vi "Keithley 6514 Limits Config.vi"(0 "Resource In":refnum<visa-resource-name>, 1 "limit 1 test (off:F)":bool, 2 "limit 2 test (off:F)":bool, 3 "Input Path for Limits (Inputs:0)":u16(ring) items=["Inputs ", "Results of Math"], 4 "pass line":dbl min=0.0 max=15.0 step=1.0, 5 "error in (no error)":T1, 6 "upper limit 1 (1)":dbl=1.0 min=-9.99999e+20 max=9.99999e+20 step=1.0 format="%.5e", 7 "upper limit 2 (1)":dbl=1.0 min=-9.99999e+20 max=9.99999e+20 step=1.0 format="%.5e", 8 "lower limit 1 (-1)":dbl=-1.0 min=-9.99999e+20 max=9.99999e+20 step=1.0 format="%.5e", 9 "lower limit 2 (-1)":dbl=-1.0 min=-9.99999e+20 max=9.99999e+20 step=1.0 format="%.5e", 10 "UL1 fail line (15)":i8=15 min=0 max=15 step=1, 11 "UL2 fail line (15)":i8=15 min=0 max=15 step=1, 12 "LL1 fail line (15)":i8=15 min=0 max=15 step=1, 13 "LL2 fail line (15)":i8=15 min=0 max=15 step=1, 15 "Check For SCPI Errors? (T)":bool=TRUE, 18 "Clear I/O Port \nWhen :INIT Sent (on:T)":bool=TRUE) -> (14 "Resource Out (dupl)":refnum<visa-resource-name>, 19 "error out":T1)   [LabVIEW 2014, in "KE6514Driver.lvlib"]
doc: "This VI is used to configure the settings for math calculation 2 Limits configuration. This involves performing limit tests on each measurement.\n\nTo read the results of the calculation, use the Limits Results VI.\n\nInput Path for Limits:\n0 = Input Signals\n1 = Result of Math\n\nLimit 1 Test:\nTRUE = On\nFALSE = Off\n\nLimit 2 Test:\nTRUE = On\nFALSE = Off\n\nPass Line: \n0 to 15\n\nUpper Limit 1:\n-9.99999e20 to +9.99999e20\n\nLower Limit 1:\n-9.99999e20 to +9.99999e20\n\nUpper Limit 2:\n-9.99999e20 to +9.99999e20\n\nLower Limit 2:\n-9.99999e20 to +9.99999e20\n\nUL1 Fail Line:\n0 to 15\n\nLL1 Fail Line:\n0 to 15\n\nUL2 Fail Line:\n0 to 15\n\nLL2 Fail Line:\n0 to 15\n\nClear I/O Port When :INIT Sent:\nTRUE = On\nFALSE = Off"
uses:
  KE6514Driver.lvlib
panel:
  # "on\noff"
  # "on\noff"
  # "on\noff"
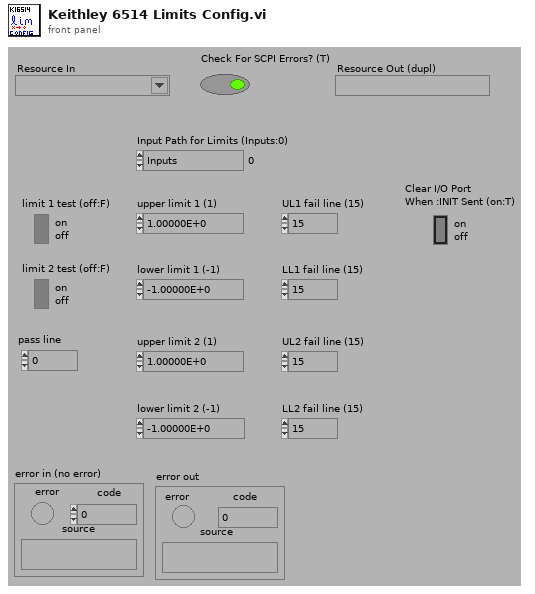
[diagram p1: front panel]
types:
  T1 = cluster{"error":bool, "code":i32, "source":string}
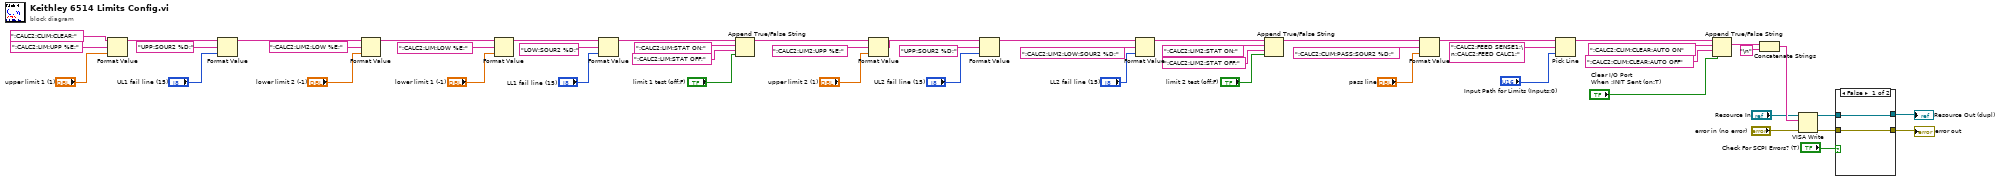
[diagram p0: block diagram]
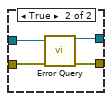
[diagram p2: hidden frame]
diagram:
  n1 = Format Value(string ("")=":CALC2:CLIM:CLEAR;", format string=":CALC2:LIM:UPP %E;", value (0)="upper limit 1 (1)") -> (output string=w1:string)
  n2 = Format Value(string ("")=w1, format string="UPP:SOUR2 %D;", value (0)="UL1 fail line (15)") -> (output string=w2:string)
  n3 = Format Value(string ("")=w2, format string=":CALC2:LIM2:LOW %E;", value (0)="lower limit 2 (-1)") -> (output string=w3:string)
  n4 = Format Value(string ("")=w3, format string=":CALC2:LIM:LOW %E;", value (0)="lower limit 1 (-1)") -> (output string=w4:string)
  n5 = Format Value(string ("")=w4, format string="LOW:SOUR2 %D;", value (0)="LL1 fail line (15)") -> (output string=w5:string)
  n6 = Append True/False String(1:"limit 1 test (off:F)", 2:":CALC2:LIM:STAT OFF;", 3:":CALC2:LIM:STAT ON;", 4:w5) -> (0:w6:string)
  n7 = Format Value(string ("")=w6, format string=":CALC2:LIM2:UPP %E;", value (0)="upper limit 2 (1)") -> (output string=w7:string)
  n8 = Format Value(string ("")=w7, format string="UPP:SOUR2 %D;", value (0)="UL2 fail line (15)") -> (output string=w8:string)
  n9 = Format Value(string ("")=w8, format string=":CALC2:LIM2:LOW:SOUR2 %D;", value (0)="LL2 fail line (15)") -> (output string=w9:string)
  n10 = Append True/False String(1:"limit 2 test (off:F)", 2:":CALC2:LIM2:STAT OFF;", 3:":CALC2:LIM2:STAT ON;", 4:w9) -> (0:w10:string)
  n11 = Format Value(string ("")=w10, format string=":CALC2:CLIM:PASS:SOUR2 %D;", value (0)="pass line") -> (output string=w11:string)
  n12 = Pick Line(string ("")=w11, multi-line string=":CALC2:FEED SENSE1;\n:CALC2:FEED CALC1;", line index="Input Path for Limits (Inputs:0)") -> (output string=w12:string)
  n13 = Append True/False String(1:"Clear I/O Port \nWhen :INIT Sent (on:T)", 2:":CALC2:CLIM:CLEAR:AUTO OFF", 3:":CALC2:CLIM:CLEAR:AUTO ON", 4:w12) -> (0:w18:string)
  n14 = Concatenate Strings(w18, "\n") -> (w22:string)
  n15 = VISA Write(VISA resource name="Resource In", write buffer=w22, error in (no error)="error in (no error)") -> (VISA resource name out=w16:refnum<visa-resource-name>, error out=w15:errorcluster)  [unwired: 1 out]
  n16 = case shown="False" "Check For SCPI Errors? (T)" {
    tunnel: w16 -> [w54 w57]
    tunnel: w15 -> [w53 w58]
    tunnel: [w54 w56] -> w13
    tunnel: [w53 w55] -> w14
    frame False {
    }
    frame True {
      n17 = call "Error Query.vi"("VISA Resource In"=w57, "error in (no error)"=w58) -> ("VISA Resource Out (dupl)"=w56:refnum<visa-resource-name>, "error out"=w55:errorcluster)  [unwired: 10 in, 2 out]
    }
  }
  "error out" <- w14
  "Resource Out (dupl)" <- w13
